vi "Configure Timebase Parameters.vi"(0 "Session Handle in":T4, 7 "Horizontal Settings":T2={"Time/div"=0.01, "Trigger Holdoff"=0.0} {"Time/div" scale=0.0001..1.0 scale format="%#_8g"}, 11 "error in (no error)":errorcluster) -> (4 "Session Handle out":T4, 8 "[Meta]SetupInfoTrigger":T1, 15 "error out":errorcluster)   [LabVIEW 2019, in "SmartScopeDriver.lvclass"]
doc: "Sets up the timebase of the smart scope."
uses:
  SmartScopeDriver.lvclass
  Typedefs/Session Handle.ctl
  Scope Driver/Typedef/Horizontal Settings.ctl
  Scope Driver/Typedef/TimeSetting.ctl
  Scope Driver/Typedef/Metadata/[Meta]SetupInfoTrigger.ctl
  SmartScopeDriver.lvclass/SmartScopeDriver.ctl
  Scope Driver/LabNation Scope Driver.lvlib
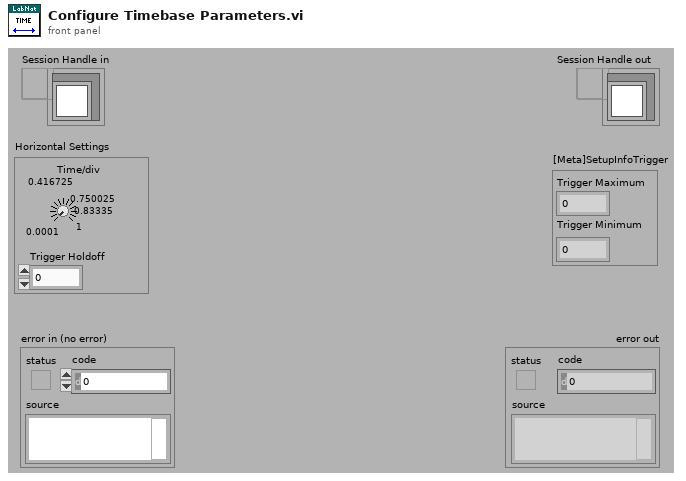
[diagram p1: front panel]
types:
  T1 = typedef "LabNation Scope Driver.lvlib/[Meta]SetupInfoTrigger.ctl" = cluster{"Trigger Maximum":dbl, "Trigger Minimum":dbl}
  T2 = typedef "LabNation Scope Driver.lvlib/Horizontal Settings.ctl" = cluster{"Time/div":T3, "Trigger Holdoff":dbl}
  T3 = typedef "LabNation Scope Driver.lvlib/TimeSetting.ctl" = dbl
  T4 = typedef "SmartScopeDriver.lvclass/Session Handle.ctl" = refnum<data-value>
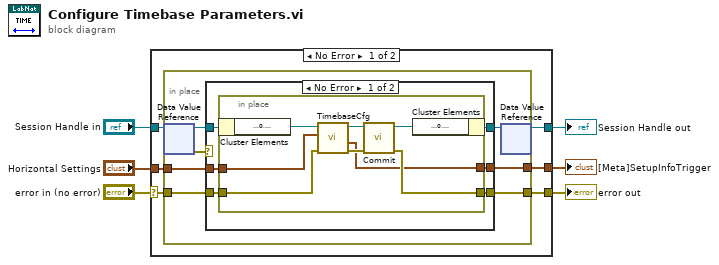
[diagram p0: block diagram]
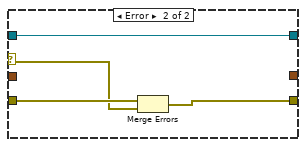
[diagram p2: hidden frame]
diagram:
  n1 = case shown="No Error" "error in (no error)" {
    selector: "error in (no error)" -> [w10 w38]
    tunnel: "Session Handle in" -> [w12 w39]
    tunnel: [w11 w39] -> w5
    tunnel: [w9 w38] -> w4
    tunnel: [w8 _] -> w2
    tunnel: "Horizontal Settings" -> [w7 _]
    frame No Error {
      n2 = in-place {
        in-place-border: w10 -> [w15]
        in-place-border: [w18] -> w9
        in-place-border: [w14] -> w8
        in-place-border: w7 -> [w13]
        n3 = in-place-dvr #1(w12) -> (w19:refnum<class "SmartScopeDriver.lvclass">, w16:errorcluster)
        n4 = case shown="No Error" w16 {
          selector: w16 -> [_ w36]
          tunnel: w19 -> [w25 w34]
          tunnel: [w24 w35] -> w18
          tunnel: [w23 w34] -> w17
          tunnel: w15 -> [w22 w37]
          tunnel: [w21 _] -> w14
          tunnel: w13 -> [w20 _]
          frame No Error {
            n5 = in-place {
              in-place-border: [w29] -> w24
              in-place-border: w22 -> [w28]
              in-place-border: [w27] -> w21
              in-place-border: w20 -> [w26]
              n6 = in-place-cluster #2(w25) -> ("reference"=w31:refnum<k24>)
              n7 = call "TimebaseCfg.vi"("error in (no error)"=w28, "Horizontal Settings"=w26, "reference in"=w31) -> ("error out"=w33:errorcluster, "[Meta]SetupInfoTrigger"=w27:T1, "reference out"=w32:refnum<k24>)  [unwired: 6 in]
              n8 = call "Commit.vi"("error in (no error)"=w33, "reference in"=w32) -> ("error out"=w29:errorcluster, "reference out"=w30:refnum<k24>)  [unwired: 8 in]
              n9 = in-place-cluster #2("reference"=w30) -> (w23:refnum<class "SmartScopeDriver.lvclass">)
            }
          }
          frame Error {
            n10 = Merge Errors(w37, w36) -> (w35:errorcluster)
          }
        }
        n11 = in-place-dvr #1(w17) -> (w11:T4)  [unwired: 1 out]
      }
    }
    frame Error {
    }
  }
  "Session Handle out" <- w5
  "error out" <- w4
  "[Meta]SetupInfoTrigger" <- w2
